vi "Stop ILCs.vi"(8 "error in (no error)":errorcluster, 11 "Model in":refnum<class "Model.lvclass">) -> (0 "error out":errorcluster, 3 "Model out":refnum<class "Model.lvclass">)   [LabVIEW 2015, in "Model.lvclass"]
uses:
  Model.lvclass
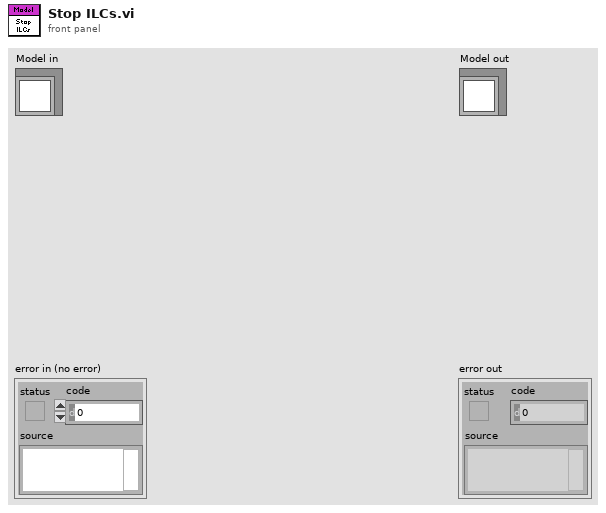
[diagram p1: front panel]
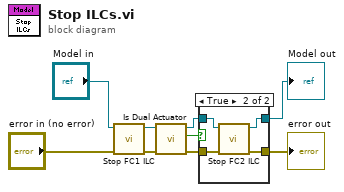
[diagram p0: block diagram]
diagram:
  n1 = call "Stop FC1 ILC.vi"("error in (no error)"="error in (no error)", "Model in"="Model in") -> ("error out"=w5:errorcluster, "Model out"=w1:refnum<class "Model.lvclass">)  [unwired: 8 in]
  n2 = call "Is Dual Actuator.vi"("error in (no error)"=w5, "Model in"=w1) -> ("error out"=w4:errorcluster, "Is Dual Actuator"=w3:bool, "Model out"=w2:refnum<class "Model.lvclass">)  [unwired: 7 in]
  n3 = case shown="True" w3 {
    tunnel: w2 -> [w11 w15]
    tunnel: [w11 w14] -> w8
    tunnel: w4 -> [w10 w13]
    tunnel: [w10 w12] -> w6
    frame False {
    }
    frame True {
      n4 = call "Stop FC2 ILC.vi"("error in (no error)"=w13, "Model in"=w15) -> ("error out"=w12:errorcluster, "Model out"=w14:refnum<class "Model.lvclass">)  [unwired: 8 in]
    }
  }
  "error out" <- w6
  "Model out" <- w8
